vi "Build Entry Assign Buffer.vi"(9 "Only Writers":bool, 10 "Name":string, 11 "Field ID":T1) -> (3 "data string":string)   [LabVIEW 2017]
uses:
  <vilib>/Rock Robotics/Network Tables/Field ID.ctl
  <vilib>/Rock Robotics/Network Tables/Make Table Operation.ctl
  <vilib>/Rock Robotics/Network Tables/Field Type.ctl
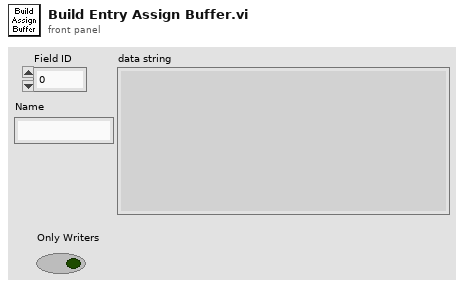
[diagram p1: front panel]
types:
  T1 = typedef "Field ID.ctl" = i32
  T2 = typedef "Field Type.ctl" = enum8{"Invalid", "Bool", "Numeric", "String", "Raw", "Boolean Array", "Numeric Array", "String Array", "RPC"}
  T3 = typedef "Make Table Operation.ctl" = enum16{"Get or Add Field", "Get Field or Add Temp", "Replace Temp ID", "Get Field ID - No Add", "Get Table Field IDs", "Get Field ID Info", "Move Field to Temp", "Validate", "Remove Field", "Remove All"}
  T4 = typedef "Field Data.ctl" = cluster{"Dbl":dbl, "String":string, "Type":T2, "Boolean":bool, "Sequence #":T5, "Flags":u8}
  T5 = typedef "Sequence.ctl" = u16
  T6 = cluster{"Type out":u8, u16, "Sequence #":T5, "Flags":u8}
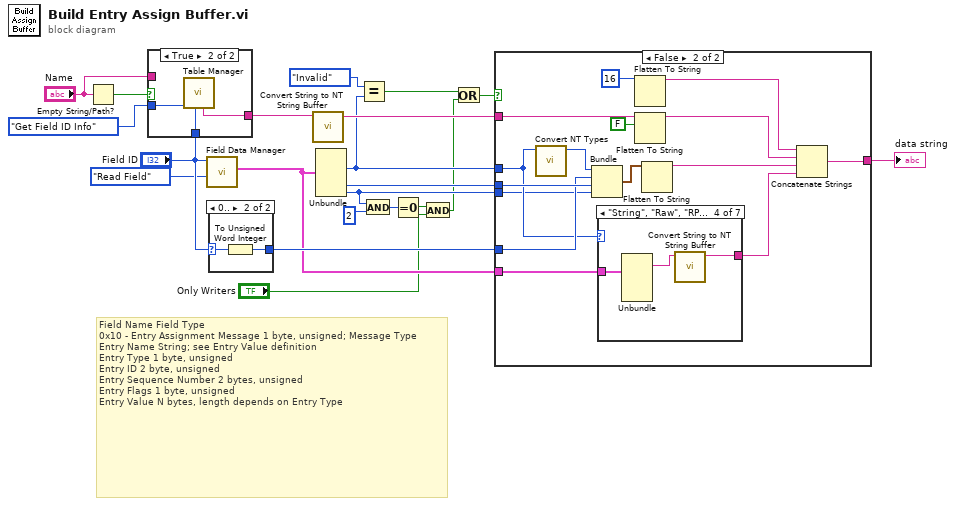
[diagram p0: block diagram]
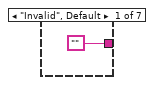
[diagram p3: hidden frame]
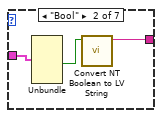
[diagram p4: hidden frame]
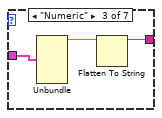
[diagram p5: hidden frame]
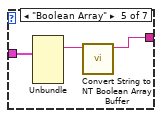
[diagram p6: hidden frame]
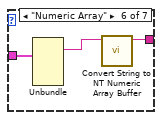
[diagram p7: hidden frame]
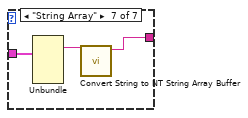
[diagram p8: hidden frame]
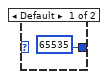
[diagram p10: hidden frame]
diagram:
  # "Field Name\tField Type\n0x10 - Entry Assignment Message\t1 byte, unsigned; Message Type\nEntry Name\tString; see Entry Value definition\nEntry Type\t1 byte, unsigned\nEntry ID\t2 byte, unsigned\nEntry Sequence Number\t2 bytes, unsigned\nEntry Flags 1 byte, unsigned\nEntry Value\tN bytes, length depends on Entry Type"
  n1 = Empty String/Path?(string/path="Name") -> (empty?=w12:bool)
  n2 = case shown="True" w12 {
    tunnel: Make_Table_Operation."Get Field ID Info" ("Operation") -> [_ w25]
    tunnel: [w22 w24] -> w20
    tunnel: "Field ID" -> [_ w23]
    tunnel: "Name" -> [w22 _]
    frame False {
    }
    frame True {
      n3 = call <vilib>:"Table Manager.vi"("Entry ID in"=w23, "Operation"=w25) -> ("Entry Name"=w24:string)  [unwired: 6 in, 3 out]
    }
  }
  n4 = call <vilib>:"Field Data Manager.vi"("Operation"=enum16{"Update Field", "Read Field"}."Read Field", "Field ID"="Field ID") -> ("Field Value Out"=w13:T4)  [unwired: 8 in, 1 out]
  n5 = case shown="0.." "Field ID" {
    selector: "Field ID" -> [_ w28]
    tunnel: [u16 65535 w27] -> w15
    frame Default {
    }
    frame 0.. {
      n6 = To Unsigned Word Integer(number=w28) -> (unsigned 16bit integer=w27:u16)
    }
  }
  n7 = call <vilib>:"Convert String to NT String Buffer.vi"("LV Buffer"=w20) -> ("NT Buffer"=w19:string)  [unwired: 10 in]
  n8 = Unbundle(w13) -> ("Type"=w10:T2, "Sequence #"=w18:T5, "Flags"=w8:u8)  [unwired: 3 out]
  n9 = Equal?(x=Field_Type."Invalid" ("Type"), y=w10) -> (x = y?=w2:bool)
  n10 = And(x=w8, y=2) -> (x .and. y?=w6:i32)
  n11 = Equal To 0?(x=w6) -> (x = 0?=w5:bool)
  n12 = And(x=w5, y="Only Writers") -> (x .and. y?=w3:bool)
  n13 = Or(x=w2, y=w3) -> (x .or. y?=w1:bool)
  n14 = case shown="False" w1 {
    tunnel: w19 -> [_ w42]
    tunnel: w18 -> [_ w37]
    tunnel: [_ w34] -> w17
    tunnel: w15 -> [_ w33]
    tunnel: w10 -> [_ w32]
    tunnel: w13 -> [_ w31]
    tunnel: w8 -> [_ w29]
    frame True {
      # "During reconnection, only explicitly written\nvariables are sent."
      # "Invalid types don't get sent to the server"
    }
    frame False {
      n15 = call <vilib>:"Convert NT Types.vi"("Type in"=w32) -> ("Type out"=w38:u8)  [unwired: 10 in]
      n16 = Bundle("Type out"=w38, w33, "Sequence #"=w37, "Flags"=w29) -> (w36:T6)  [unwired: 1 in]
      n17 = case shown="\"String\", \"Raw\", \"RPC\"" w32 {
        tunnel: w31 -> [_ w47 w50 w53 w56 w59 w62]
        tunnel: ["" w45 w48 w51 w54 w57 w60] -> w30
        frame "Invalid", Default {
        }
        frame "Bool" {
          n18 = Unbundle(w47) -> ("Boolean"=w46:bool)  [unwired: 5 out]
          n19 = call <vilib>:"Convert NT Boolean to LV String.vi"("Boolean"=w46) -> ("string"=w45:string)  [unwired: 10 in]
        }
        frame "Numeric" {
          n20 = Unbundle(w50) -> ("Dbl"=w49:dbl)  [unwired: 5 out]
          n21 = Flatten To String(anything=w49) -> (data string=w48:string)  [unwired: 3 in, 2 out]
        }
        frame "String", "Raw", "RPC" {
          n22 = Unbundle(w53) -> ("String"=w52:string)  [unwired: 5 out]
          n23 = call <vilib>:"Convert String to NT String Buffer.vi"("LV Buffer"=w52) -> ("NT Buffer"=w51:string)  [unwired: 10 in]
        }
        frame "Boolean Array" {
          n24 = Unbundle(w56) -> ("String"=w55:string)  [unwired: 5 out]
          n25 = call <vilib>:"Convert String to NT Boolean Array Buffer.vi"("LV Buffer"=w55) -> ("NT Buffer"=w54:string)  [unwired: 10 in]
        }
        frame "Numeric Array" {
          n26 = Unbundle(w59) -> ("String"=w58:string)  [unwired: 5 out]
          n27 = call <vilib>:"Convert String to NT Numeric Array Buffer.vi"("LV Buffer"=w58) -> ("NT Buffer"=w57:string)  [unwired: 10 in]
        }
        frame "String Array" {
          n28 = Unbundle(w62) -> ("String"=w61:string)  [unwired: 5 out]
          n29 = call <vilib>:"Convert String to NT String Array Buffer.vi"("LV Buffer"=w61) -> ("NT Buffer"=w60:string)  [unwired: 10 in]
        }
      }
      n30 = Flatten To String(anything=u8 16 ("bytes to read")) -> (data string=w40:string)  [unwired: 3 in, 2 out]
      n31 = Flatten To String(anything=w42, prepend array or string size? (T)=FALSE) -> (data string=w39:string)  [unwired: 2 in, 2 out]
      n32 = Flatten To String(anything=w36) -> (data string=w35:string)  [unwired: 3 in, 2 out]
      n33 = Concatenate Strings(w40, w39, w35, w30) -> (w34:string)
    }
  }
  "data string" <- w17
